vi "Destroy Messenger.vi"(8 "error in (no error)":errorcluster, 11 "Network Client Reference In":refnum<data-value>) -> (0 "error out":errorcluster)   [LabVIEW 2020, in "Network Messenger.lvlib" / "Network Messenger.lvclass"]
uses:
  <vilib>/gpm_packages/@cs/Network-interface/Source/Network Messenger/Network Messenger.lvclass
  <vilib>/gpm_packages/@cs/Network-interface/Source/Network Messenger/Network Messenger.lvclass/Network Messenger.ctl
  <vilib>/ActorFramework/Message Enqueuer/Message Enqueuer.lvclass/Message Enqueuer.ctl
  <vilib>/ActorFramework/Message Enqueuer/Enqueue.vi
  <vilib>/ActorFramework/Stop Msg/Stop Msg.lvclass
  C:/Program Files/National Instruments/LabVIEW 2020/vi.lib/ActorFramework/Message/Message.lvclass
  <vilib>/ActorFramework/Message Priority Queue/Priority Enqueue.vi
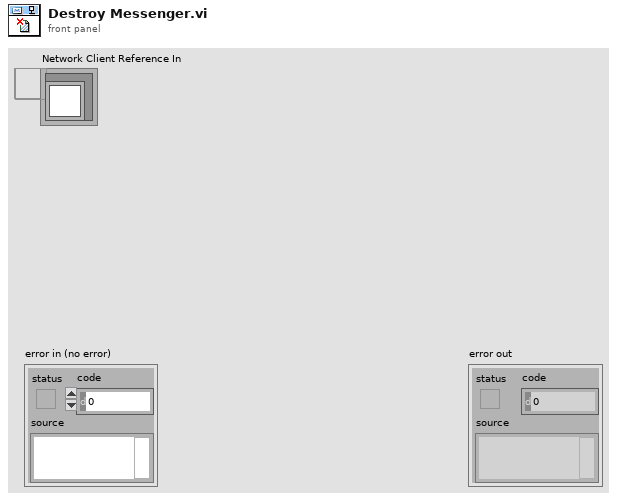
[diagram p1: front panel]
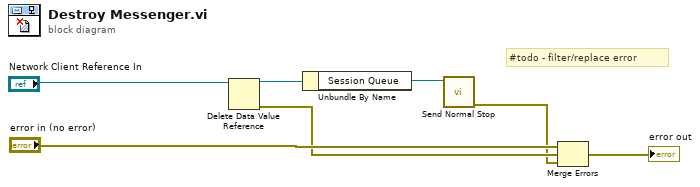
[diagram p0: block diagram]
diagram:
  # "#todo - filter/replace error"
  n1 = Delete Data Value Reference(data value reference="Network Client Reference In") -> (data value=w3:refnum<class "Network Messenger.lvclass">, error out=w4:errorcluster)  [unwired: 1 in]
  n2 = Unbundle By Name(w3) -> ("Session Queue"=w2:refnum<class "Message Enqueuer.lvclass">)
  n3 = call <vilib>:"Send Normal Stop.vi"("Message Enqueuer"=w2) -> ("error out"=w1:errorcluster)  [unwired: 10 in]
  n4 = Merge Errors("error in (no error)", w4, w1) -> (→"error out":errorcluster)
